vi "ACDC_Config.vi"(8 "error in (no error)":errorcluster, 9 "Input Config Array":T1[](array[typedef])=[0, 0, 0, 0, 0, 0, 0, 0, 0, 0, 0, 0, 0, 0, 0, 0, 0, 0, 0, 0, 0, 0, 0, 0, 0, 0, 0, 0, 0, 0, 0, 0] items=["AC Coupled", "DC Coupled", "IEPE AC Coupled"], 10 "Data Rate [S/s]":u32) -> (0 "error out":errorcluster)   [LabVIEW 2017, in "BOP_VibAPI_2.lvlib"]
uses:
  <vilib>/addons/InsightCM/Devices/Shared/Cms/Fpga/Acquisition/source/subVIs/VibAPI_2/BOP_VibAPI_2.lvlib
  <vilib>/LabVIEW Targets/FPGA/cRIO/shared/nicrio_ModuleControls/nicrio_cRIO-9232_ConfigModeRing.ctl
  <vilib>/rvi/eio/common/nirviEmuTemplatePropertySet_errors.vi
  <vilib>/eio/EIOPropertyNode/EIOPropertyNode.xnode
  <vilib>/LabVIEW Targets/FPGA/cRIO/shared/nicrio_ModuleControls/nicrio_cRIO-9232_DataRatesRing2.ctl
  <vilib>/rvi/eio/common/nirviEmuTemplatePropertyGet_errors.vi
  <vilib>/rvi/eio/common/nirviEmuTemplatePropertyGet_noerrors.vi
  <vilib>/rvi/eio/common/nirviEmuTemplatePropertySet_noerrors.vi
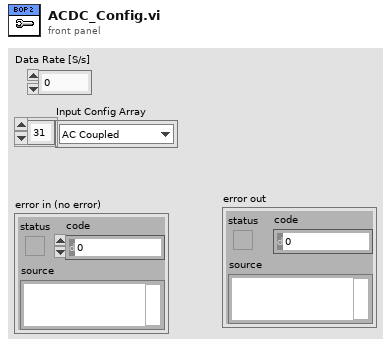
[diagram p1: front panel]
types:
  T1 = typedef "nicrio_cRIO-9232_ConfigModeRing.ctl" = u8
  T2 = typedef "nicrio_cRIO-9232_DataRatesRing2.ctl" = u8
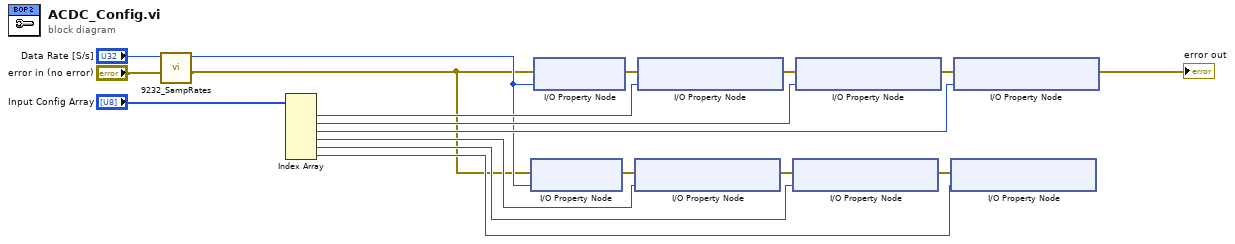
[diagram p0: block diagram]
diagram:
  n1 = call <vilib>:"9232_SampRates.vi"("error in (no error)"="error in (no error)", "Data Rate [S/s]"="Data Rate [S/s]") -> ("error out"=w3:errorcluster, "Data Rate"=w4:T2)  [unwired: 8 in]
  n2 = Index Array(array="Input Config Array") -> (element #1=w10:T1, element #2=w9:T1, element #3=w5:T1, element #4=w8:T1, element #5=w7:T1, element #6=w6:T1)  [unwired: 6 in]
  n3 = xnode "I/O Property Node"("error in"=w3, "Data Rate"=w4) -> ("error out"=w11:errorcluster)  [unwired: 1 in, 1 out]
  n4 = xnode "I/O Property Node"("error in"=w3, "Data Rate"=w4) -> ("error out"=w12:errorcluster)  [unwired: 1 in, 1 out]
  n5 = xnode "I/O Property Node"("error in"=w11, "Input Configuration"=w8) -> ("error out"=w15:errorcluster)  [unwired: 1 in, 1 out]
  n6 = xnode "I/O Property Node"("error in"=w12, "Input Configuration"=w10) -> ("error out"=w13:errorcluster)  [unwired: 1 in, 1 out]
  n7 = xnode "I/O Property Node"("error in"=w15, "Input Configuration"=w7) -> ("error out"=w16:errorcluster)  [unwired: 1 in, 1 out]
  n8 = xnode "I/O Property Node"("error in"=w13, "Input Configuration"=w9) -> ("error out"=w14:errorcluster)  [unwired: 1 in, 1 out]
  n9 = xnode "I/O Property Node"("error in"=w16, "Input Configuration"=w6) -> ()  [unwired: 1 in, 2 out]
  n10 = xnode "I/O Property Node"("error in"=w14, "Input Configuration"=w5) -> ("error out"=→"error out":errorcluster)  [unwired: 1 in, 1 out]
